vi "1B_Combination_Digitizer_Driver.vi"(0 "Mode":T1(ring), 1 "Horizontal Settings":T2={"number of records"=1, "reference position"=50.0, "min record length"=50000, "min sample rate"=200000.0, "enforce realtime"=FALSE, "maximum input frequency"=0.0} {"maximum input frequency" format="%.2f"; "min sample rate" step=1000000.0; "reference position" format="%.1f"; "number of records" step=1}, 2 "Vertical Settings":T4={"vertical coupling"=enum."DC", "probe attenuation"=20.0, "vertical range"=120.0, "vertical offset"=0.0} {"vertical offset" format="%.4f"; "vertical range" format="%.2f"; "probe attenuation" format="%.1f"}, 3 "Trigger settings":T3={"trigger level"=30.0, "trigger type"=enum."Edge", "Trigger Source"=enum."Channel 0", "Trigger Slope"=enum."Positive"} {"trigger level" format="%.2f"}, 5 "Channel Name":string="0", 11 "error in":errorcluster) -> (6 "Waveform Array":waveform(dbl)[](array[waveform]), 8 "Ch1_Plot":dbl[](array[numeric]), 15 "error out":errorcluster)   [LabVIEW 2010]
uses:
  <instrlib>/niScope/Controls/niScope trigger slope.ctl
  <instrlib>/niScope/Controls/niScope trigger source.ctl
  <instrlib>/niScope/Controls/niScope export destinations.ctl
  <instrlib>/niScope/Controls/niScope exportable signals.ctl
  <instrlib>/niScope/Controls/niScope trigger source digital.ctl
  <instrlib>/niScope/Configure/Trigger/niScope Configure Trigger Edge.vi
  <instrlib>/niScope/Configure/Trigger/niScope Configure Trigger Digital.vi
  <instrlib>/niScope/Configure/Trigger/niScope Configure Trigger Immediate.vi
  <instrlib>/niScope/Acquire/niScope Multi Read Cluster.vi
  <instrlib>/niScope/Acquire/Fetch/niScope Multi Fetch Cluster.vi
panel:
  in  "resource name Dig1":refnum<k15>="PXI1Slot6"
  in  "resource name Dig2":refnum<k15>="PXI1Slot4"
  out "Waveform":T5(graph)
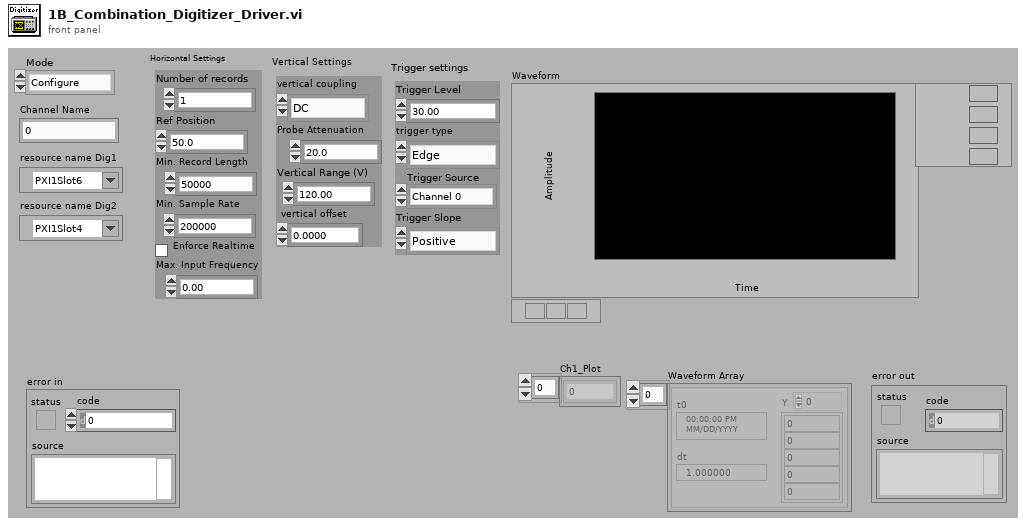
[diagram p1: front panel]
types:
  T1 = enum16{"Configure", "Read", "TriggerRead", "Close", "Init"}
  T2 = cluster{"number of records":i32, "reference position":dbl, "min record length":i32, "min sample rate":dbl, "enforce realtime":bool, "maximum input frequency":dbl}
  T3 = cluster{"trigger level":dbl, "trigger type":enum16{"Edge", "Digital", "Immediate"}, "Trigger Source":enum8{"Immediate", "Channel 0", "Channel 1", "Channel 2", "Channel 3", "Channel 4", "Channel 5", "Channel 6", "Channel 7", "External TRIG", "Software Trigger", "RTSI 0", "RTSI 1", "RTSI 2", "RTSI 3", "RTSI 4", "RTSI 5", "RTSI 6", "PFI 0", "PFI 1", "PFI 2", "PXI Star Trigger"}, "Trigger Slope":enum16{"Positive", "Negative"}}
  T4 = cluster{"vertical coupling":enum16{"AC", "DC", "Ground"}, "probe attenuation":dbl, "vertical range":dbl, "vertical offset":dbl}
  T5 = cluster{"relativeInitialX":dbl, "xIncrement":dbl, "wfm":dbl[]}[]
  T6 = typedef "niScope trigger source.ctl" = string
  T7 = typedef "niScope trigger source digital.ctl" = string
  T8 = typedef "niScope export destinations.ctl" = string
  T9 = cluster{"Dig1 Channels":string, "Channel1 Scale":dbl, "Dig1 Used":bool, "Dig1 Ref":refnum<k15>, "min record length":i32, "Dig2 Channels":string, "Dig2 Used":bool, "Dig2 Ref":refnum<k15>, "trigger type":enum16{"Edge", "Digital", "Immediate"}}
  T10 = enum8{"Immediate", "Channel 0", "Channel 1", "Channel 2", "Channel 3", "Channel 4", "Channel 5", "Channel 6", "Channel 7", "External TRIG", "Software Trigger", "RTSI 0", "RTSI 1", "RTSI 2", "RTSI 3", "RTSI 4", "RTSI 5", "RTSI 6", "PFI 0", "PFI 1", "PFI 2", "PXI Star Trigger"}
  T11 = typedef "niScope exportable signals.ctl" = u16
  T12 = typedef "niScope trigger slope.ctl" = i32
  T13 = cluster{"relativeInitialX":dbl, "xIncrement":dbl, "wfm":dbl[]}
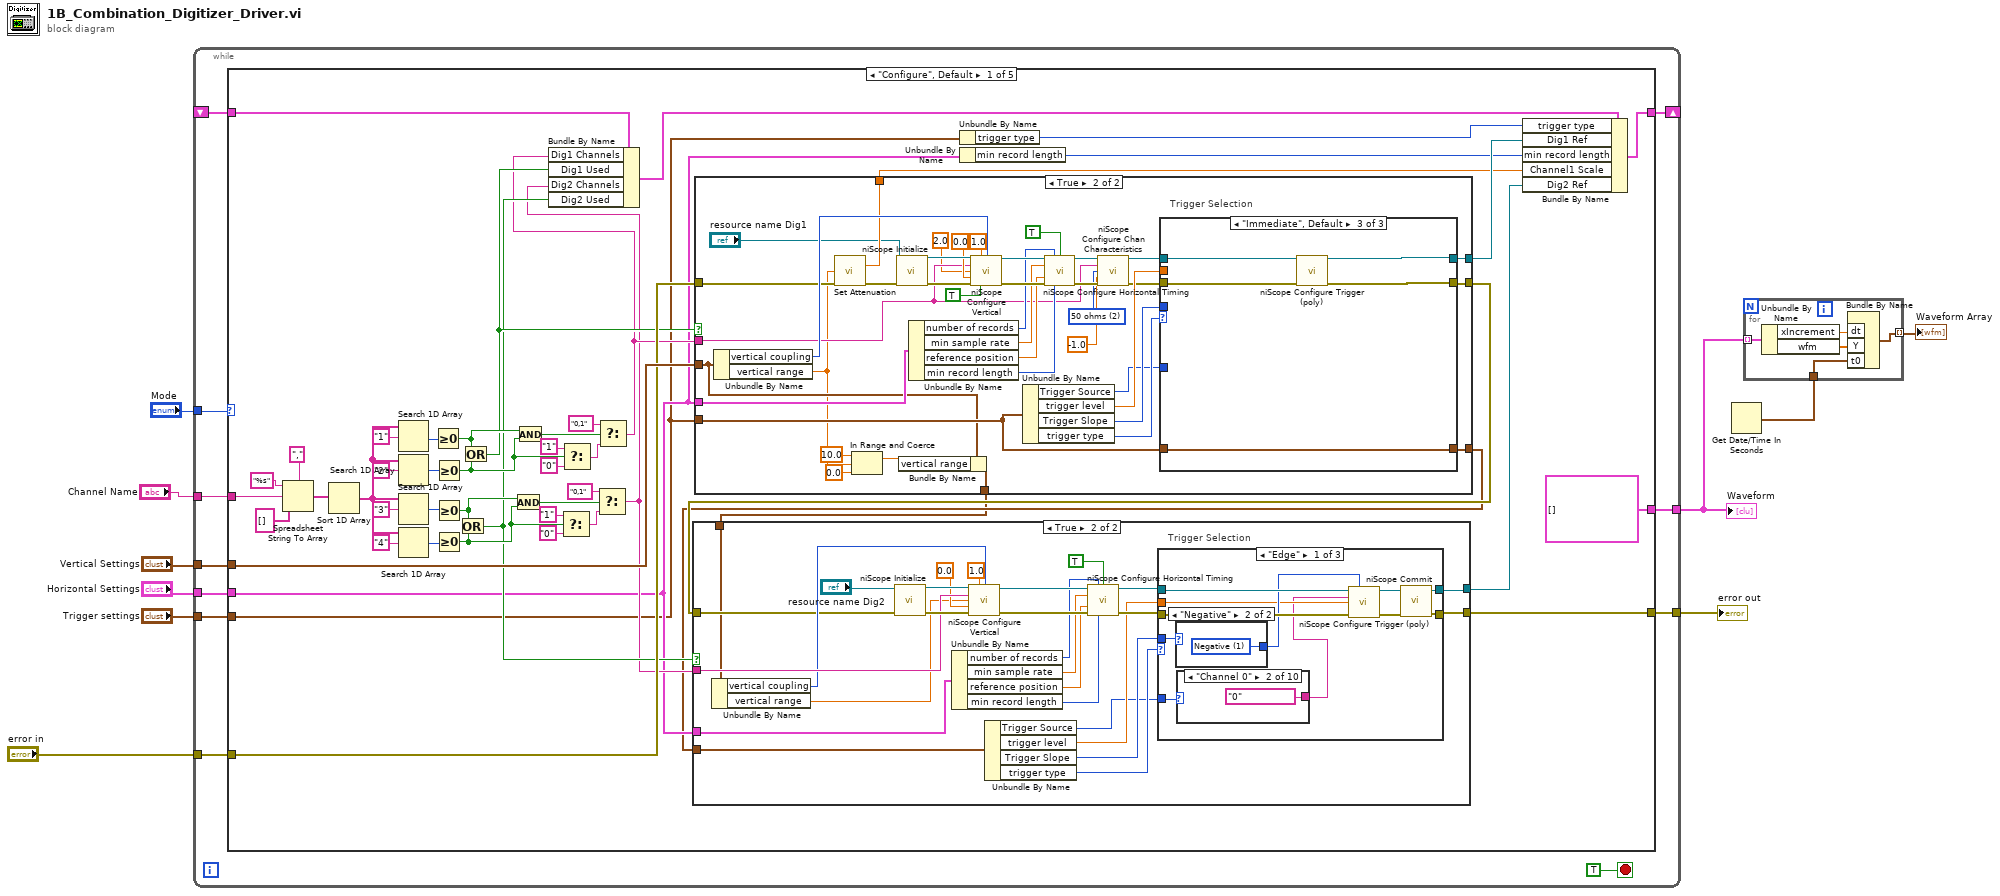
[diagram p0: block diagram]
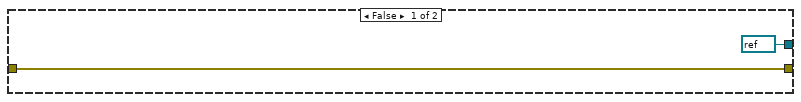
[diagram p2: hidden frame]
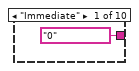
[diagram p3: hidden frame]
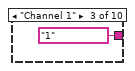
[diagram p4: hidden frame]
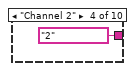
[diagram p5: hidden frame]
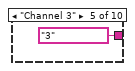
[diagram p6: hidden frame]
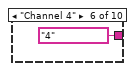
[diagram p7: hidden frame]
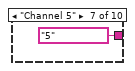
[diagram p8: hidden frame]
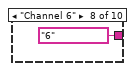
[diagram p9: hidden frame]
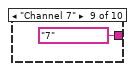
[diagram p10: hidden frame]
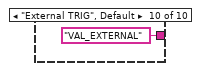
[diagram p11: hidden frame]
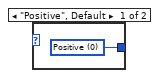
[diagram p12: hidden frame]
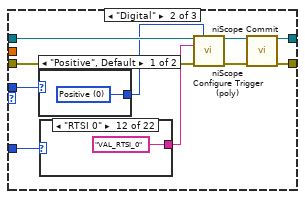
[diagram p13: hidden frame]
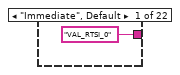
[diagram p14: hidden frame]
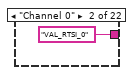
[diagram p15: hidden frame]
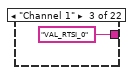
[diagram p16: hidden frame]
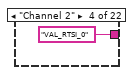
[diagram p17: hidden frame]
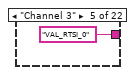
[diagram p18: hidden frame]
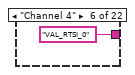
[diagram p19: hidden frame]
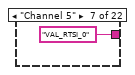
[diagram p20: hidden frame]
diagram:
  n1 = while {
    tunnel: "Mode" -> [w20]
    shift-right: [w14] -> _
    shift-left: _ -> [w19]
    tunnel: "error in" -> [w13]
    tunnel: "Channel Name" -> [w18]
    tunnel: "Vertical Settings" -> [w17]
    tunnel: "Horizontal Settings" -> [w16]
    tunnel: "Trigger settings" -> [w15]
    tunnel: [w12] -> w5
    tunnel: [w11] -> w3
    stop <- TRUE stop-if-true
    n2 = case shown="\"Configure\", Default" w20 {
      tunnel: w19 -> [w38 w315 w418 w445 w494]
      tunnel: w18 -> [w42 _ _ _ _]
      tunnel: w17 -> [w41 _ _ _ _]
      tunnel: w16 -> [w28 _ _ _ _]
      tunnel: w15 -> [w25 _ _ _ _]
      tunnel: [w40 w315 w418 w445 T9 {"Dig1 Channels"="", "Channel1 Scale"=0.0, "Dig1 Used"=FALSE, "Dig1 Ref"="", "min record length"=0, "Dig2 Channels"="", "Dig2 Used"=FALSE, "Dig2 Ref"="", "trigger type"=enum."Immediate"}] -> w14
      tunnel: w13 -> [w39 w321 w421 w451 w497]
      tunnel: [w33 w326 w424 w456 w500] -> w12
      tunnel: [T5 [] w313 T5 [] w444 T5 []] -> w11
      frame "Configure", Default {
        n3 = Spreadsheet String To Array(delimiter (Tab)=",", format string="%s", spreadsheet string=w42, array type (2D Dbl)=string[] []) -> (array=w67:string[])
        n4 = Sort 1D Array(array=w67) -> (sorted array=w66:string[])
        n5 = Search 1D Array(1D array=w66, element="1") -> (index of element=w61:i32)  [unwired: 1 in]
        n6 = Search 1D Array(1D array=w66, element="2") -> (index of element=w58:i32)  [unwired: 1 in]
        n7 = Search 1D Array(1D array=w66, element="3") -> (index of element=w59:i32)  [unwired: 1 in]
        n8 = Search 1D Array(1D array=w66, element="4") -> (index of element=w60:i32)  [unwired: 1 in]
        n9 = Greater Or Equal To 0?(x=w61) -> (x >= 0?=w57:bool)
        n10 = Greater Or Equal To 0?(x=w58) -> (x >= 0?=w53:bool)
        n11 = Greater Or Equal To 0?(x=w59) -> (x >= 0?=w56:bool)
        n12 = Greater Or Equal To 0?(x=w60) -> (x >= 0?=w44:bool)
        n13 = Or(x=w56, y=w44) -> (x .or. y?=w31:bool)
        n14 = Or(x=w57, y=w53) -> (x .or. y?=w32:bool)
        n15 = And(x=w56, y=w44) -> (x .and. y?=w45:bool)
        n16 = And(x=w57, y=w53) -> (x .and. y?=w55:bool)
        n17 = Select(t="1", s=w44, f="0") -> (s? t:f=w47:string)
        n18 = Select(t="1", s=w53, f="0") -> (s? t:f=w51:string)
        n19 = Select(t="0,1", s=w45, f=w47) -> (s? t:f=w29:string)
        n20 = Select(t="0,1", s=w55, f=w51) -> (s? t:f=w30:string)
        n21 = Bundle By Name(cluster=w38, "Dig1 Channels"=w30, "Dig1 Used"=w32, "Dig2 Channels"=w29, "Dig2 Used"=w31) -> (w37:T9)
        n22 = case shown="True" w32 {
          tunnel: [w165 w203] -> w43
          tunnel: w39 -> [w165 w200]
          tunnel: w30 -> [_ w174]
          tunnel: w41 -> [w161 w181]
          tunnel: w28 -> [_ w195]
          tunnel: w25 -> [w162 w183]
          tunnel: [refnum<k15> refnum ("instrument handle out") w189] -> w36
          tunnel: [1.0 ("Gain Multiplier") w187] -> w34
          tunnel: [w162 w182] -> w23
          tunnel: [w161 w180] -> w22
          frame False {
          }
          frame True {
            w173 = u32 2 items=["1 mega ohm"=0, "50 ohms"=2] ("input impedance")
            n23 = Unbundle By Name(w181) -> ("vertical coupling"=w202:enum16{"AC", "DC", "Ground"}, "vertical range"=w169:dbl)
            n24 = call "Set Attenuation.vi"("vertical range"=w169, "error in"=w200) -> ("Gain Multiplier"=w187:dbl, "error out"=w199:errorcluster)  [unwired: 11 in, 1 out]
            n25 = In Range and Coerce(upper limit=10.0, x=w169, lower limit=0.0) -> (coerced(x)=w166:dbl)  [unwired: 1 out]
            n26 = call <instrlib>:"niScope Initialize.vi"("resource name"="resource name Dig1", "error in"=w199) -> ("instrument handle"=w205:refnum<k15>, "error out"=w204:errorcluster)  [unwired: 12 in]
            n27 = Bundle By Name(cluster=w181, "vertical range"=w166) -> (w180:T4)
            n28 = Unbundle By Name(w195) -> ("number of records"=w194:i32, "min sample rate"=w193:dbl, "reference position"=w192:dbl, "min record length"=w191:i32)
            n29 = call <instrlib>:"niScope Configure Vertical.vi"("instrument handle"=w205, "probe attenuation"=1.0, "vertical coupling"=w202, "channels"=w174, "vertical range"=2.0, "vertical offset"=0.0, "error in"=w204, "channel enabled"=TRUE) -> ("instrument handle out"=w197:refnum<k15>, "error out"=w196:errorcluster)  [unwired: 6 in]
            n30 = Unbundle By Name(w183) -> ("Trigger Source"=w184:T10, "trigger level"=w190:dbl, "Trigger Slope"=w185:enum16{"Positive", "Negative"}, "trigger type"=w186:enum16{"Edge", "Digital", "Immediate"})
            n31 = call <instrlib>:"niScope Configure Horizontal Timing.vi"("instrument handle"=w197, "number of records"=w194, "enforce realtime"=TRUE, "min sample rate"=w193, "reference position"=w192, "error in"=w196, "min record length"=w191) -> ("instrument handle out"=w178:refnum<k15>, "error out"=w176:errorcluster)  [unwired: 7 in]
            n32 = call <instrlib>:"niScope Configure Chan Characteristics.vi"("instrument handle"=w178, "channels"=w174, "input impedance"=w173, "maximum input frequency"=-1.0, "error in"=w176) -> ("instrument handle out"=w177:refnum<k15>, "error out"=w175:errorcluster)  [unwired: 9 in]
            n33 = case "Trigger Selection" shown="\"Immediate\", Default" w186 {
              tunnel: w175 -> [w207 w279 w308]
              tunnel: [w212 w272 w305] -> w203
              tunnel: w177 -> [w209 w278 w307]
              tunnel: [w213 w273 w306] -> w189
              tunnel: w184 -> [w217 w275 _]
              tunnel: w190 -> [w218 _ _]
              tunnel: w185 -> [w220 w277 _]
              tunnel: w183 -> [w211 w271 w304]
              tunnel: [w210 w271 w304] -> w182
              frame "Edge" {
                n34 = case shown="\"Channel 0\"" w217 {
                  tunnel: [T6 "0" ("trigger source") T6 "0" ("trigger source") T6 "1" ("trigger source") T6 "2" ("trigger source") T6 "3" ("trigger source") T6 "4" ("trigger source") T6 "5" ("trigger source") T6 "6" ("trigger source") T6 "7" ("trigger source") T6 "VAL_EXTERNAL" ("trigger source")] -> w216
                  tunnel: w211 -> [w223 _ _ w243 w247 w251 w255 w259 w263 w267]
                  tunnel: [w223 T3 {"trigger level"=0.0, "trigger type"=enum."Digital", "Trigger Source"=enum."RTSI 0", "Trigger Slope"=enum."Positive"} ("Trigger settings") T3 {"trigger level"=0.0, "trigger type"=enum."Digital", "Trigger Source"=enum."RTSI 0", "Trigger Slope"=enum."Positive"} ("Trigger settings") w243 w247 w251 w255 w259 w263 w267] -> w210
                  tunnel: w209 -> [w222 w228 w236 w242 w246 w250 w254 w258 w262 w266]
                  tunnel: [w222 w226 w235 w242 w246 w250 w254 w258 w262 w266] -> w208
                  tunnel: w207 -> [w221 w227 w234 w241 w245 w249 w253 w257 w261 w265]
                  tunnel: [w221 w225 w233 w241 w245 w249 w253 w257 w261 w265] -> w206
                  frame "Immediate" {
                  }
                  frame "Channel 0" {
                    w229 = T11 1 items=["None"=0, "Start Trigger"=2, "Advance Trigger"=5, "Reference Trigger"=1, "End of Record Event"=4, "End of Acquisition Event"=3, "Ready for Start Event"=7, "Ready for Advance Event"=6, "Ready for Reference Event"=10, "Reference Clock"=100, "Sample Clock"=101, "5 Volt Power"=13] ("signal")
                    n35 = call <instrlib>:"niScope Export Signal.vi"("instrument handle"=w228, "signal"=w229, "output terminal"=T8 "VAL_RTSI_0", "error in"=w227) -> ("instrument handle out"=w226:refnum<k15>, "error out"=w225:errorcluster)  [unwired: 10 in]
                  }
                  frame "Channel 1" {
                    w237 = T11 1 items=["None"=0, "Start Trigger"=2, "Advance Trigger"=5, "Reference Trigger"=1, "End of Record Event"=4, "End of Acquisition Event"=3, "Ready for Start Event"=7, "Ready for Advance Event"=6, "Ready for Reference Event"=10, "Reference Clock"=100, "Sample Clock"=101, "5 Volt Power"=13] ("signal")
                    n36 = call <instrlib>:"niScope Export Signal.vi"("instrument handle"=w236, "signal"=w237, "output terminal"=T8 "VAL_RTSI_0", "error in"=w234) -> ("instrument handle out"=w235:refnum<k15>, "error out"=w233:errorcluster)  [unwired: 10 in]
                  }
                  frame "Channel 2" {
                  }
                  frame "Channel 3" {
                  }
                  frame "Channel 4" {
                  }
                  frame "Channel 5" {
                  }
                  frame "Channel 6" {
                  }
                  frame "Channel 7" {
                  }
                  frame "External TRIG", Default {
                  }
                }
                n37 = case shown="\"Positive\", Default" w220 {
                  tunnel: [w269 w270] -> w219
                  frame "Positive", Default {
                    w269 = T12 0 items=["Positive", "Negative"] ("trigger slope")
                  }
                  frame "Negative" {
                    w270 = T12 1 items=["Positive", "Negative"] ("trigger slope")
                  }
                }
                n38 = call-poly <instrlib>:"niScope Configure Trigger (poly).vi"("instrument handle"=w208, "trigger slope"=w219, "trigger source"=w216, "trigger level"=w218, "error in"=w206) -> ("instrument handle out"=w215:refnum<k15>, "error out"=w214:errorcluster)  [unwired: 9 in]
                n39 = call <instrlib>:"niScope Commit.vi"("instrument handle"=w215, "error in"=w214) -> ("instrument handle out"=w213:refnum<k15>, "error out"=w212:errorcluster)  [unwired: 12 in]
              }
              frame "Digital" {
                n40 = case shown="\"Negative\"" w277 {
                  tunnel: [w302 w303] -> w276
                  frame "Positive", Default {
                    w302 = T12 0 items=["Positive", "Negative"] ("trigger slope")
                  }
                  frame "Negative" {
                    w303 = T12 1 items=["Positive", "Negative"] ("trigger slope")
                  }
                }
                n41 = case shown="\"PXI Star Trigger\"" w275 {
                  tunnel: [T7 "VAL_RTSI_0" ("trigger source") T7 "VAL_RTSI_0" ("trigger source") T7 "VAL_RTSI_0" ("trigger source") T7 "VAL_RTSI_0" ("trigger source") T7 "VAL_RTSI_0" ("trigger source") T7 "VAL_RTSI_0" ("trigger source") T7 "VAL_RTSI_0" ("trigger source") T7 "VAL_RTSI_0" ("trigger source") T7 "VAL_RTSI_0" ("trigger source") T7 "VAL_RTSI_0" ("trigger source") T7 "VAL_RTSI_0" ("trigger source") T7 "VAL_RTSI_0" ("trigger source") T7 "VAL_RTSI_1" ("trigger source") T7 "VAL_RTSI_2" ("trigger source") T7 "VAL_RTSI_3" ("trigger source") T7 "VAL_RTSI_4" ("trigger source") T7 "VAL_RTSI_5" ("trigger source") T7 "VAL_RTSI_6" ("trigger source") T7 "VAL_PFI_0" ("trigger source") T7 "VAL_PFI_1" ("trigger source") T7 "VAL_PFI_2" ("trigger source") T7 "VAL_PXI_STAR" ("trigger source")] -> w274
                  frame "Immediate", Default {
                  }
                  frame "Channel 0" {
                  }
                  frame "Channel 1" {
                  }
                  frame "Channel 2" {
                  }
                  frame "Channel 3" {
                  }
                  frame "Channel 4" {
                  }
                  frame "Channel 5" {
                  }
                  frame "Channel 6" {
                  }
                  frame "Channel 7" {
                  }
                  frame "External TRIG" {
                  }
                  frame "Software Trigger" {
                  }
                  frame "RTSI 0" {
                  }
                  frame "RTSI 1" {
                  }
                  frame "RTSI 2" {
                  }
                  frame "RTSI 3" {
                  }
                  frame "RTSI 4" {
                  }
                  frame "RTSI 5" {
                  }
                  frame "RTSI 6" {
                  }
                  frame "PFI 0" {
                  }
                  frame "PFI 1" {
                  }
                  frame "PFI 2" {
                  }
                  frame "PXI Star Trigger" {
                  }
                }
                n42 = call-poly <instrlib>:"niScope Configure Trigger (poly).vi"("instrument handle"=w278, "trigger slope"=w276, "trigger source"=w274, "error in"=w279) -> ("instrument handle out"=w273:refnum<k15>, "error out"=w272:errorcluster)  [unwired: 10 in]
              }
              frame "Immediate", Default {
                n43 = call-poly <instrlib>:"niScope Configure Trigger (poly).vi"("instrument handle"=w307, "error in"=w308) -> ("instrument handle out"=w306:refnum<k15>, "error out"=w305:errorcluster)  [unwired: 12 in]
              }
            }
          }
        }
        n44 = case shown="True" w31 {
          tunnel: [w72 w80] -> w33
          tunnel: w43 -> [w72 w85]
          tunnel: w29 -> [_ w97]
          tunnel: w28 -> [_ w91]
          tunnel: w23 -> [_ w86]
          tunnel: [refnum<k15> refnum ("instrument handle out") w81] -> w35
          tunnel: w22 -> [_ w74]
          frame False {
          }
          frame True {
            n45 = Unbundle By Name(w74) -> ("vertical coupling"=w96:enum16{"AC", "DC", "Ground"}, "vertical range"=w84:dbl)
            n46 = call <instrlib>:"niScope Initialize.vi"("resource name"="resource name Dig2", "error in"=w85) -> ("instrument handle"=w99:refnum<k15>, "error out"=w98:errorcluster)  [unwired: 12 in]
            n47 = Unbundle By Name(w91) -> ("number of records"=w90:i32, "min sample rate"=w89:dbl, "reference position"=w88:dbl, "min record length"=w87:i32)
            n48 = call <instrlib>:"niScope Configure Vertical.vi"("instrument handle"=w99, "probe attenuation"=1.0, "vertical coupling"=w96, "channels"=w97, "vertical range"=w84, "vertical offset"=0.0, "error in"=w98) -> ("instrument handle out"=w93:refnum<k15>, "error out"=w92:errorcluster)  [unwired: 7 in]
            n49 = Unbundle By Name(w86) -> ("Trigger Source"=w75:T10, "trigger level"=w78:dbl, "Trigger Slope"=w76:enum16{"Positive", "Negative"}, "trigger type"=w77:enum16{"Edge", "Digital", "Immediate"})
            n50 = call <instrlib>:"niScope Configure Horizontal Timing.vi"("instrument handle"=w93, "number of records"=w90, "enforce realtime"=TRUE, "min sample rate"=w89, "reference position"=w88, "error in"=w92, "min record length"=w87) -> ("instrument handle out"=w82:refnum<k15>, "error out"=w79:errorcluster)  [unwired: 7 in]
            n51 = case "Trigger Selection" shown="\"Edge\"" w77 {
              tunnel: w79 -> [w110 w132 w160]
              tunnel: [w100 w123 w157] -> w80
              tunnel: w82 -> [w109 w131 w159]
              tunnel: [w102 w124 w158] -> w81
              tunnel: w75 -> [w105 w128 _]
              tunnel: w78 -> [w106 _ _]
              tunnel: w76 -> [w108 w130 _]
              frame "Edge" {
                n52 = case shown="\"Negative\"" w108 {
                  tunnel: [w121 w122] -> w107
                  frame "Positive", Default {
                    w121 = T12 0 items=["Positive", "Negative"] ("trigger slope")
                  }
                  frame "Negative" {
                    w122 = T12 1 items=["Positive", "Negative"] ("trigger slope")
                  }
                }
                n53 = case shown="\"Channel 0\"" w105 {
                  tunnel: [T6 "0" ("trigger source") T6 "0" ("trigger source") T6 "1" ("trigger source") T6 "2" ("trigger source") T6 "3" ("trigger source") T6 "4" ("trigger source") T6 "5" ("trigger source") T6 "6" ("trigger source") T6 "7" ("trigger source") T6 "VAL_EXTERNAL" ("trigger source")] -> w104
                  frame "Immediate" {
                  }
                  frame "Channel 0" {
                  }
                  frame "Channel 1" {
                  }
                  frame "Channel 2" {
                  }
                  frame "Channel 3" {
                  }
                  frame "Channel 4" {
                  }
                  frame "Channel 5" {
                  }
                  frame "Channel 6" {
                  }
                  frame "Channel 7" {
                  }
                  frame "External TRIG", Default {
                  }
                }
                n54 = call-poly <instrlib>:"niScope Configure Trigger (poly).vi"("instrument handle"=w109, "trigger slope"=w107, "trigger source"=w104, "trigger level"=w106, "error in"=w110) -> ("instrument handle out"=w103:refnum<k15>, "error out"=w101:errorcluster)  [unwired: 9 in]
                n55 = call <instrlib>:"niScope Commit.vi"("instrument handle"=w103, "error in"=w101) -> ("instrument handle out"=w102:refnum<k15>, "error out"=w100:errorcluster)  [unwired: 12 in]
              }
              frame "Digital" {
                n56 = case shown="\"Positive\", Default" w130 {
                  tunnel: [w155 w156] -> w129
                  frame "Positive", Default {
                    w155 = T12 0 items=["Positive", "Negative"] ("trigger slope")
                  }
                  frame "Negative" {
                    w156 = T12 1 items=["Positive", "Negative"] ("trigger slope")
                  }
                }
                n57 = case shown="\"RTSI 0\"" w128 {
                  tunnel: [T7 "VAL_RTSI_0" ("trigger source") T7 "VAL_RTSI_0" ("trigger source") T7 "VAL_RTSI_0" ("trigger source") T7 "VAL_RTSI_0" ("trigger source") T7 "VAL_RTSI_0" ("trigger source") T7 "VAL_RTSI_0" ("trigger source") T7 "VAL_RTSI_0" ("trigger source") T7 "VAL_RTSI_0" ("trigger source") T7 "VAL_RTSI_0" ("trigger source") T7 "VAL_RTSI_0" ("trigger source") T7 "VAL_RTSI_0" ("trigger source") T7 "VAL_RTSI_0" ("trigger source") T7 "VAL_RTSI_1" ("trigger source") T7 "VAL_RTSI_2" ("trigger source") T7 "VAL_RTSI_3" ("trigger source") T7 "VAL_RTSI_4" ("trigger source") T7 "VAL_RTSI_5" ("trigger source") T7 "VAL_RTSI_6" ("trigger source") T7 "VAL_PFI_0" ("trigger source") T7 "VAL_PFI_1" ("trigger source") T7 "VAL_PFI_2" ("trigger source") T7 "VAL_PXI_STAR" ("trigger source")] -> w127
                  frame "Immediate", Default {
                  }
                  frame "Channel 0" {
                  }
                  frame "Channel 1" {
                  }
                  frame "Channel 2" {
                  }
                  frame "Channel 3" {
                  }
                  frame "Channel 4" {
                  }
                  frame "Channel 5" {
                  }
                  frame "Channel 6" {
                  }
                  frame "Channel 7" {
                  }
                  frame "External TRIG" {
                  }
                  frame "Software Trigger" {
                  }
                  frame "RTSI 0" {
                  }
                  frame "RTSI 1" {
                  }
                  frame "RTSI 2" {
                  }
                  frame "RTSI 3" {
                  }
                  frame "RTSI 4" {
                  }
                  frame "RTSI 5" {
                  }
                  frame "RTSI 6" {
                  }
                  frame "PFI 0" {
                  }
                  frame "PFI 1" {
                  }
                  frame "PFI 2" {
                  }
                  frame "PXI Star Trigger" {
                  }
                }
                n58 = call-poly <instrlib>:"niScope Configure Trigger (poly).vi"("instrument handle"=w131, "trigger slope"=w129, "trigger source"=w127, "error in"=w132) -> ("instrument handle out"=w126:refnum<k15>, "error out"=w125:errorcluster)  [unwired: 10 in]
                n59 = call <instrlib>:"niScope Commit.vi"("instrument handle"=w126, "error in"=w125) -> ("instrument handle out"=w124:refnum<k15>, "error out"=w123:errorcluster)  [unwired: 12 in]
              }
              frame "Immediate", Default {
                n60 = call-poly <instrlib>:"niScope Configure Trigger (poly).vi"("instrument handle"=w159, "error in"=w160) -> ("instrument handle out"=w158:refnum<k15>, "error out"=w157:errorcluster)  [unwired: 12 in]
              }
            }
          }
        }
        n61 = Unbundle By Name(w25) -> ("trigger type"=w24:enum16{"Edge", "Digital", "Immediate"})
        n62 = Unbundle By Name(w28) -> ("min record length"=w27:i32)
        n63 = Bundle By Name(cluster=w37, "trigger type"=w24, "Dig1 Ref"=w36, "min record length"=w27, "Channel1 Scale"=w34, "Dig2 Ref"=w35) -> (w40:T9)
      }
      frame "Read" {
        n64 = Unbundle By Name(w315) -> ("trigger type"=w310:enum16{"Edge", "Digital", "Immediate"}, "Dig1 Used"=w325:bool, "Dig1 Ref"=w324:refnum<k15>, "Dig1 Channels"=w323:string, "min record length"=w322:i32, "Channel1 Scale"=w316:dbl)
        n65 = Unbundle By Name(w315) -> ("trigger type"=w309:enum16{"Edge", "Digital", "Immediate"}, "Dig2 Used"=w320:bool, "Dig2 Ref"=w319:refnum<k15>, "Dig2 Channels"=w318:string, "min record length"=w317:i32)
        n66 = case shown="True" w325 {
          tunnel: w323 -> [_ w389]
          tunnel: w321 -> [w383 w387]
          tunnel: w324 -> [_ w390]
          tunnel: [w383 w385] -> w327
          tunnel: [T5 [] ("waveform") w386] -> w328
          tunnel: w322 -> [_ w388]
          tunnel: w310 -> [_ w384]
          frame False {
          }
          frame True {
            n67 = case shown="\"Digital\", Default" w384 {
              tunnel: w390 -> [w397 w407]
              tunnel: w389 -> [w396 w406]
              tunnel: w388 -> [w395 w405]
              tunnel: w387 -> [w394 w404]
              tunnel: [w392 w399] -> w386
              tunnel: [w391 w402] -> w385
              frame "Immediate" {
                n68 = call-poly <instrlib>:"niScope Read (poly).vi"("timeout"=10.0, "error in"=w394, "numSamples"=w395, "channels"=w396, "instrument handle"=w397) -> ("error out"=w391:errorcluster, "waveform"=w392:T5)  [unwired: 3 in, 2 out]
              }
              frame "Digital", Default {
                n69 = call-poly <instrlib>:"niScope Fetch (poly).vi"("timeout"=10.0, "error in"=w404, "numSamples"=w405, "channels"=w406, "instrument handle"=w407) -> ("error out"=w401:errorcluster, "waveform"=w400:T5, "instrument handle out"=w398:refnum<k15>)  [unwired: 3 in, 1 out]
                n70 = case shown="Error" w401 {
                  tunnel: w401 -> [w408 w414]
                  tunnel: [w408 w411] -> w402
                  tunnel: w400 -> [w409 _]
                  tunnel: [w409 T5 [{"relativeInitialX"=0.0, "xIncrement"=0.0, "wfm"=[]}, {"relativeInitialX"=0.0, "xIncrement"=0.0, "wfm"=[]}] ("waveform")] -> w399
                  tunnel: w398 -> [_ w410]
                  frame No Error {
                  }
                  frame Error {
                    n71 = call <vilib>:"Clear Errors.vi"("error in (no error)"=w414) -> ("error out"=w412:errorcluster)  [unwired: 6 in]
                    n72 = call <instrlib>:"niScope Abort.vi"("instrument handle"=w410, "error in"=w412) -> ("error out"=w411:errorcluster)  [unwired: 12 in, 1 out]
                  }
                }
              }
            }
          }
        }
        n73 = case shown="True" w320 {
          tunnel: w318 -> [_ w354]
          tunnel: w327 -> [w350 w352]
          tunnel: w319 -> [_ w355]
          tunnel: w317 -> [_ w353]
          tunnel: [w350 w357] -> w326
          tunnel: [T5 [] ("waveform") w356] -> w331
          tunnel: w309 -> [_ w351]
          frame False {
          }
          frame True {
            n74 = case shown="\"Digital\", Default" w351 {
              tunnel: w355 -> [w364 w374]
              tunnel: w354 -> [w363 w373]
              tunnel: w353 -> [w362 w372]
              tunnel: w352 -> [w361 w371]
              tunnel: [w359 w367] -> w356
              tunnel: [w358 w368] -> w357
              frame "Immediate" {
                n75 = call-poly <instrlib>:"niScope Read (poly).vi"("timeout"=10.0, "error in"=w361, "numSamples"=w362, "channels"=w363, "instrument handle"=w364) -> ("error out"=w358:errorcluster, "waveform"=w359:T5)  [unwired: 3 in, 2 out]
              }
              frame "Digital", Default {
                n76 = call-poly <instrlib>:"niScope Fetch (poly).vi"("timeout"=10.0, "error in"=w371, "numSamples"=w372, "channels"=w373, "instrument handle"=w374) -> ("error out"=w366:errorcluster, "waveform"=w369:T5, "instrument handle out"=w365:refnum<k15>)  [unwired: 3 in, 1 out]
                n77 = case shown="Error" w366 {
                  tunnel: w366 -> [w375 w381]
                  tunnel: [w375 w377] -> w368
                  tunnel: w369 -> [w376 _]
                  tunnel: [w376 T5 [{"relativeInitialX"=0.0, "xIncrement"=0.0, "wfm"=[]}, {"relativeInitialX"=0.0, "xIncrement"=0.0, "wfm"=[]}] ("waveform")] -> w367
                  tunnel: w365 -> [_ w379]
                  frame No Error {
                  }
                  frame Error {
                    n78 = call <vilib>:"Clear Errors.vi"("error in (no error)"=w381) -> ("error out"=w378:errorcluster)  [unwired: 6 in]
                    n79 = call <instrlib>:"niScope Abort.vi"("instrument handle"=w379, "error in"=w378) -> ("error out"=w377:errorcluster)  [unwired: 12 in, 1 out]
                  }
                }
              }
            }
          }
        }
        n80 = Greater?(x=w316, y=1.0) -> (0:w330:bool)
        n81 = case shown="True" w330 {
          tunnel: w328 -> [w334 w348]
          tunnel: w316 -> [_ w335]
          tunnel: w331 -> [w333 w341]
          tunnel: [w332 w340] -> w313
          frame False {
            n82 = Build Array (concatenate)(w334, w333) -> (w332:T5)
          }
          frame True {
            # "Add scaling from TEGAM, if used"
            n83 = Index Array(array=w348, index #1=0 ("index"), index #2=1 ("index")) -> (element #1=w345:T13, element #2=w337:T13)
            n84 = Unbundle By Name(w345) -> ("wfm"=w347:dbl[])
            n85 = Unbundle By Name(w337) -> ("wfm"=w339:dbl[])
            n86 = Multiply(x=w347, y=w335) -> (x*y=w344:dbl[])
            n87 = Multiply(x=w339, y=w335) -> (x*y=w338:dbl[])
            n88 = Bundle By Name(cluster=w345, "wfm"=w344) -> (w342:T13)
            n89 = Bundle By Name(cluster=w337, "wfm"=w338) -> (w336:T13)
            n90 = Build Array (concatenate)(w342, w336, w341) -> (w340:T5)
          }
        }
        n91 = Index Array(array=w313, index=0) -> (element=w312:T13)
        n92 = Unbundle By Name(w312) -> ("wfm"=→"Ch1_Plot":dbl[])
      }
      frame "Init" {
        n93 = Unbundle By Name(w418) -> ("trigger type"=w417:enum16{"Edge", "Digital", "Immediate"}, "Dig1 Used"=w423:bool, "Dig1 Ref"=w422:refnum<k15>)
        n94 = Unbundle By Name(w418) -> ("trigger type"=w416:enum16{"Edge", "Digital", "Immediate"}, "Dig2 Used"=w420:bool, "Dig2 Ref"=w419:refnum<k15>)
        n95 = case shown="True" w423 {
          tunnel: w421 -> [w435 w438]
          tunnel: w422 -> [_ w439]
          tunnel: [w435 w437] -> w425
          tunnel: w417 -> [_ w436]
          frame False {
          }
          frame True {
            n96 = case shown="\"Digital\", Default" w436 {
              tunnel: w439 -> [_ w442]
              tunnel: w438 -> [w440 w441]
              tunnel: [w440 w443] -> w437
              frame "Immediate" {
              }
              frame "Digital", Default {
                n97 = call <instrlib>:"niScope Initiate Acquisition.vi"("instrument handle"=w442, "error in"=w441) -> ("error out"=w443:errorcluster)  [unwired: 12 in, 1 out]
              }
            }
          }
        }
        n98 = case shown="True" w420 {
          tunnel: w425 -> [w426 w428]
          tunnel: w419 -> [_ w429]
          tunnel: [w426 w430] -> w424
          tunnel: w416 -> [_ w427]
          frame False {
          }
          frame True {
            n99 = case shown="\"Digital\", Default" w427 {
              tunnel: w429 -> [_ w433]
              tunnel: w428 -> [w431 w432]
              tunnel: [w431 w434] -> w430
              frame "Immediate" {
              }
              frame "Digital", Default {
                n100 = call <instrlib>:"niScope Initiate Acquisition.vi"("instrument handle"=w433, "error in"=w432) -> ("error out"=w434:errorcluster)  [unwired: 12 in, 1 out]
              }
            }
          }
        }
      }
      frame "TriggerRead" {
        n101 = Unbundle By Name(w445) -> ("Dig1 Used"=w455:bool, "Dig1 Ref"=w454:refnum<k15>, "Dig1 Channels"=w453:string, "min record length"=w452:i32, "Channel1 Scale"=w446:dbl)
        n102 = Unbundle By Name(w445) -> ("Dig2 Used"=w450:bool, "Dig2 Ref"=w449:refnum<k15>, "Dig2 Channels"=w448:string, "min record length"=w447:i32)
        n103 = case shown="True" w455 {
          tunnel: w453 -> [_ w490]
          tunnel: w451 -> [w485 w491]
          tunnel: w454 -> [_ w489]
          tunnel: [w485 w486] -> w457
          tunnel: [T5 [] ("waveform") w488] -> w458
          tunnel: w452 -> [_ w487]
          frame False {
          }
          frame True {
            n104 = call-poly <instrlib>:"niScope Read (poly).vi"("error in"=w491, "numSamples"=w487, "channels"=w490, "instrument handle"=w489) -> ("error out"=w486:errorcluster, "waveform"=w488:T5)  [unwired: 4 in, 2 out]
          }
        }
        n105 = case shown="True" w450 {
          tunnel: w448 -> [_ w482]
          tunnel: w457 -> [w477 w483]
          tunnel: w449 -> [_ w481]
          tunnel: w447 -> [_ w480]
          tunnel: [w477 w478] -> w456
          tunnel: [T5 [] ("waveform") w479] -> w461
          frame False {
          }
          frame True {
            n106 = call-poly <instrlib>:"niScope Read (poly).vi"("error in"=w483, "numSamples"=w480, "channels"=w482, "instrument handle"=w481) -> ("error out"=w478:errorcluster, "waveform"=w479:T5)  [unwired: 4 in, 2 out]
          }
        }
        n107 = Greater?(x=w446, y=1.0) -> (0:w460:bool)
        n108 = case shown="True" w460 {
          tunnel: w458 -> [w464 w475]
          tunnel: w446 -> [_ w467]
          tunnel: w461 -> [w463 w466]
          tunnel: [w462 w465] -> w444
          frame False {
            n109 = Build Array (concatenate)(w464, w463) -> (w462:T5)
          }
          frame True {
            # "Add scaling from TEGAM, if used"
            n110 = Index Array(array=w475, index #1=0 ("index"), index #2=1 ("index")) -> (element #1=w472:T13, element #2=w469:T13)
            n111 = Unbundle By Name(w472) -> ("wfm"=w474:dbl[])
            n112 = Multiply(x=w474, y=w467) -> (x*y=w471:dbl[])
            n113 = Bundle By Name(cluster=w472, "wfm"=w471) -> (w468:T13)
            n114 = Build Array (concatenate)(w468, w469, w466) -> (w465:T5)
          }
        }
      }
      frame "Close" {
        n115 = Unbundle By Name(w494) -> ("Dig1 Used"=w499:bool, "Dig1 Ref"=w498:refnum<k15>)
        n116 = Unbundle By Name(w494) -> ("Dig2 Used"=w496:bool, "Dig2 Ref"=w495:refnum<k15>)
        n117 = case shown="True" w499 {
          tunnel: w497 -> [w506 w507]
          tunnel: w498 -> [_ w508]
          tunnel: [w506 w509] -> w501
          frame False {
          }
          frame True {
            n118 = call <instrlib>:"niScope Close.vi"("instrument handle"=w508, "error in"=w507) -> ("error out"=w509:errorcluster)  [unwired: 13 in]
          }
        }
        n119 = case shown="True" w496 {
          tunnel: w501 -> [w502 w504]
          tunnel: w495 -> [_ w503]
          tunnel: [w502 w505] -> w500
          frame False {
          }
          frame True {
            n120 = call <instrlib>:"niScope Close.vi"("instrument handle"=w503, "error in"=w504) -> ("error out"=w505:errorcluster)  [unwired: 13 in]
          }
        }
      }
    }
  }
  "error out" <- w5
  "Waveform" <- w3
  n121 = Get Date/Time In Seconds() -> (seconds since 1Jan1904=w1:timestamp)
  n122 = for {
    tunnel: w3 -> [w514] mode=indexing
    tunnel: [w511] -> w2 mode=indexing
    tunnel: w1 -> [w510]
    n123 = Unbundle By Name(w514) -> ("xIncrement"=w513:dbl, "wfm"=w512:dbl[])
    n124 = Bundle By Name("dt"=w513, "Y"=w512, "t0"=w510) -> (w511:waveform(dbl))  [unwired: 1 in]
  }
  "Waveform Array" <- w2
